vi "_fix_linux_palette_path_issue.vi"   [LabVIEW 2017]
uses:
  <vilib>/Palette API/Palette Menu/Public Type Define/Palette type.ctl
  <vilib>/Palette API/Palette Menu/Palette Menu.lvlib
  _Shared/CSM Shared.lvlib
types:
  T1 = typedef "Palette Menu.lvlib/Palette type.ctl" = i32
  T2 = typedef "Palette Menu.lvlib/Palette Data.ctl" = cluster{"display name":string, "view format":T3, "palette width":i16, "items":T4, "256 color icon":picture, "B&W color icon":picture, "help information":T6, "palette description":string, "synchronize information":T7}
  T3 = typedef "Palette Menu.lvlib/View Format.ctl" = u16
  T4 = typedef "Palette Menu.lvlib/Items.ctl" = T5[]
  T5 = typedef "Palette Menu.lvlib/Item.ctl" = cluster{"item path":path, "library path (.lvlib)":path, "use default lvlib palette":bool, "short name":string, "place VI contents":bool, "hide synchronized item":bool, "reserve spot for synch item":bool, "configure when placing VI contents":bool}
  T6 = typedef "Palette Menu.lvlib/Help Info.ctl" = cluster{"help tag":string, "help file path ":path}
  T7 = typedef "Palette Menu.lvlib/Synchronize Info.ctl" = cluster{"synchronize with directory":bool, "synchronize directory path":path}
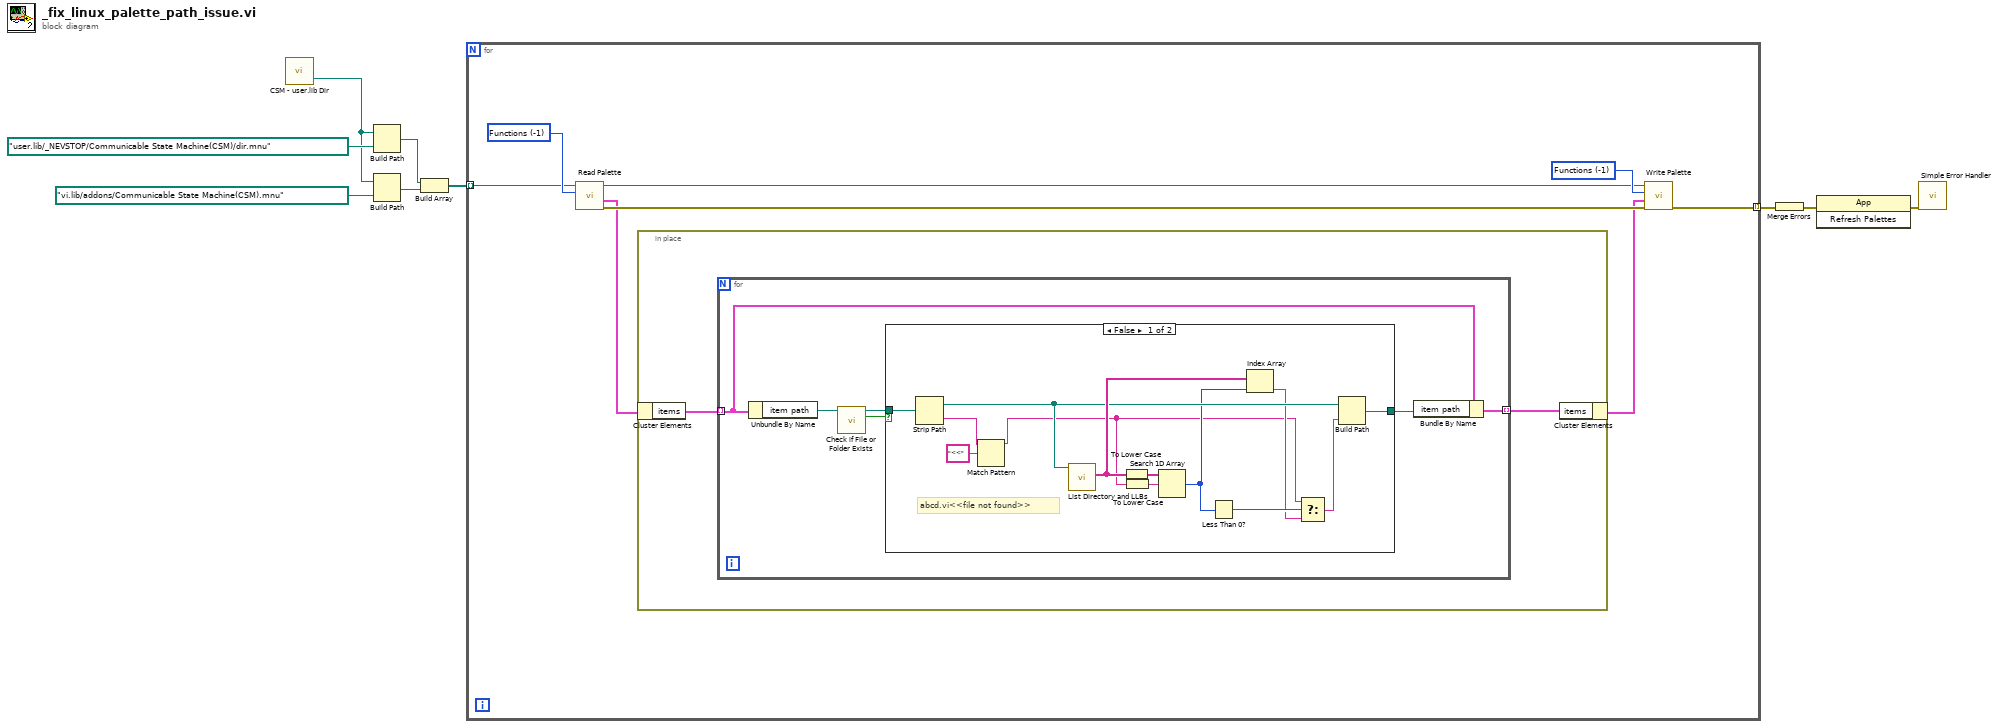
[diagram p0: block diagram]
diagram:
  n1 = call "CSM - user.lib Dir.vi"() -> ("<LabVIEW>"=w6:path)  [unwired: 2 in, 1 out]
  n2 = Build Path(base path=w6, name or relative path=path "user.lib/_NEVSTOP/Communicable State Machine(CSM)/dir.mnu") -> (appended path=w4:path)
  n3 = Build Path(base path=w6, name or relative path=path "vi.lib/addons/Communicable State Machine(CSM).mnu") -> (appended path=w5:path)
  n4 = Build Array(w4, w5) -> (w3:path[])
  n5 = for {
    tunnel: [w11] -> w8 mode=indexing
    tunnel: w3 -> [w10] mode=indexing
    w14 = T1 -1 items=["Functions"=-1, "Controls"=-2] ("palette type")
    w17 = T1 -1 items=["Functions"=-1, "Controls"=-2] ("palette type")
    n6 = call <vilib>:"Read Palette.vi"("palette type"=w14, "palette path"=w10) -> ("error out"=w16:errorcluster, "palette data"=w13:T2, "duplicate palette path"=w15:path)  [unwired: 2 in, 5 out]
    n7 = in-place {
      n8 = in-place-cluster #1(w13) -> ("items"=w19:T4)
      n9 = for {
        tunnel: w19 -> [w22] mode=indexing
        tunnel: [w21] -> w18 mode=indexing
        n10 = Unbundle By Name(w22) -> ("item path"=w25:path)
        n11 = call <vilib>:"Check if File or Folder Exists.vi"("path"=w25) -> ("file or folder exists?"=w23:bool, "dup path"=w24:path)  [unwired: 8 in, 1 out]
        n12 = case shown="False" w23 {
          tunnel: w24 -> [w38 w39]
          tunnel: [w33 w39] -> w20
          frame False {
            # "abcd.vi<<file not found>>"
            n13 = Strip Path(path=w38) -> (stripped path=w34:path, name=w28:string)
            n14 = Match Pattern(string=w28, regular expression="<<") -> (before substring=w27:string)  [unwired: 1 in, 3 out]
            n15 = call <vilib>:"List Directory and LLBs.vi"("Folder Path"=w34) -> ("Files sans LLBs"=w35:string[])  [unwired: 2 in, 8 out]
            n16 = To Lower Case(string=w35) -> (all lower case string=w37:string[])
            n17 = To Lower Case(string=w27) -> (all lower case string=w36:string)
            n18 = Search 1D Array(1D array=w37, element=w36) -> (index of element=w32:i32)  [unwired: 1 in]
            n19 = Less Than 0?(x=w32) -> (x < 0?=w31:bool)
            n20 = Index Array(array=w35, index=w32) -> (element=w30:string)
            n21 = Select(t=w27, s=w31, f=w30) -> (s? t:f=w29:string)
            n22 = Build Path(base path=w34, name or relative path=w29) -> (appended path=w33:path)
          }
          frame True {
          }
        }
        n23 = Bundle By Name(cluster=w22, "item path"=w20) -> (w21:T5)
      }
      n24 = in-place-cluster #1("items"=w18) -> (w12:T2)
    }
    n25 = call <vilib>:"Write Palette.vi"("error in (no error)"=w16, "palette data"=w12, "palette type"=w17, "palette path"=w15) -> ("error out"=w11:errorcluster)  [unwired: 1 in, 6 out]
  }
  n26 = Merge Errors(w8) -> (w2:errorcluster)
  n27 = invoke class="App" method="Refresh Palettes"(error in=w2) -> (error out=w1:errorcluster)  [unwired: 2 in, 2 out]
  n28 = call <vilib>:"Simple Error Handler.vi"("error in (no error)"=w1) -> ()  [unwired: 1 in, 8 out]
